vi "cross_talk).vi"(9 "Array":u8[](array[numeric]), 10 "Rising Index 2":i32[](array[numeric]), 11 "Rising Index":i32[](array[numeric])) -> (0 "data 2":cluster{"x":dbl, "y":dbl}[](array[cluster]) {"y" format="%.2f"; "x" format="%.2f"}, 1 "data":cluster{"x":dbl, "y":dbl}[](array[cluster]) {"y" format="%.2f"; "x" format="%.2f"}, 2 "x/y 2":dbl, 3 "x/y":dbl)   [LabVIEW 2012]
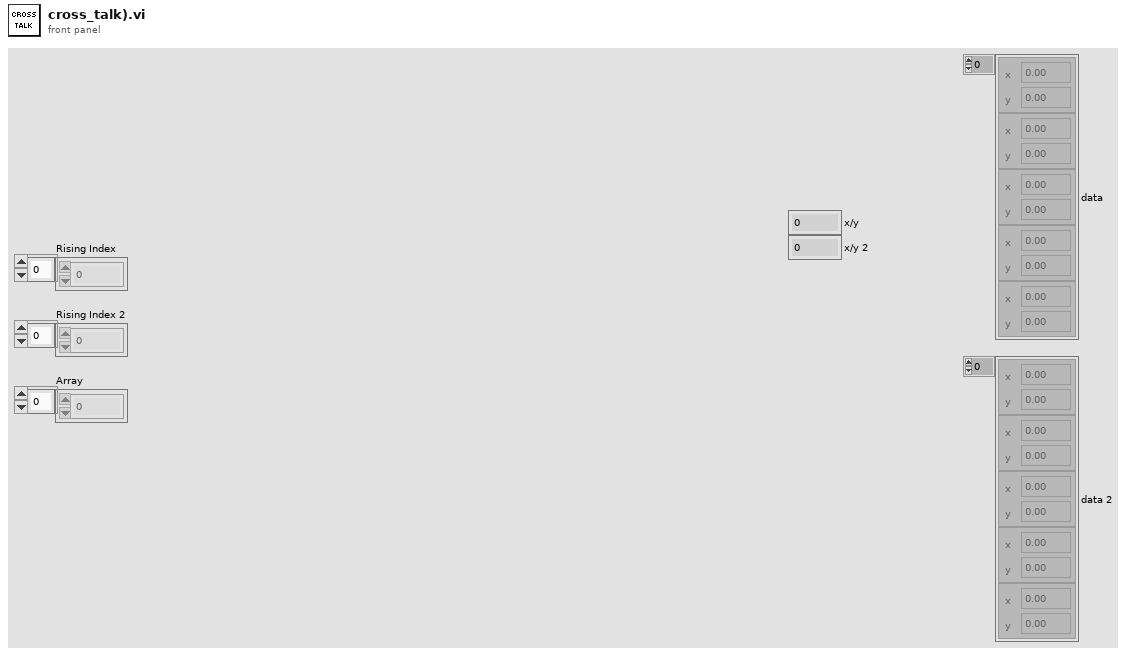
[diagram p1: front panel]
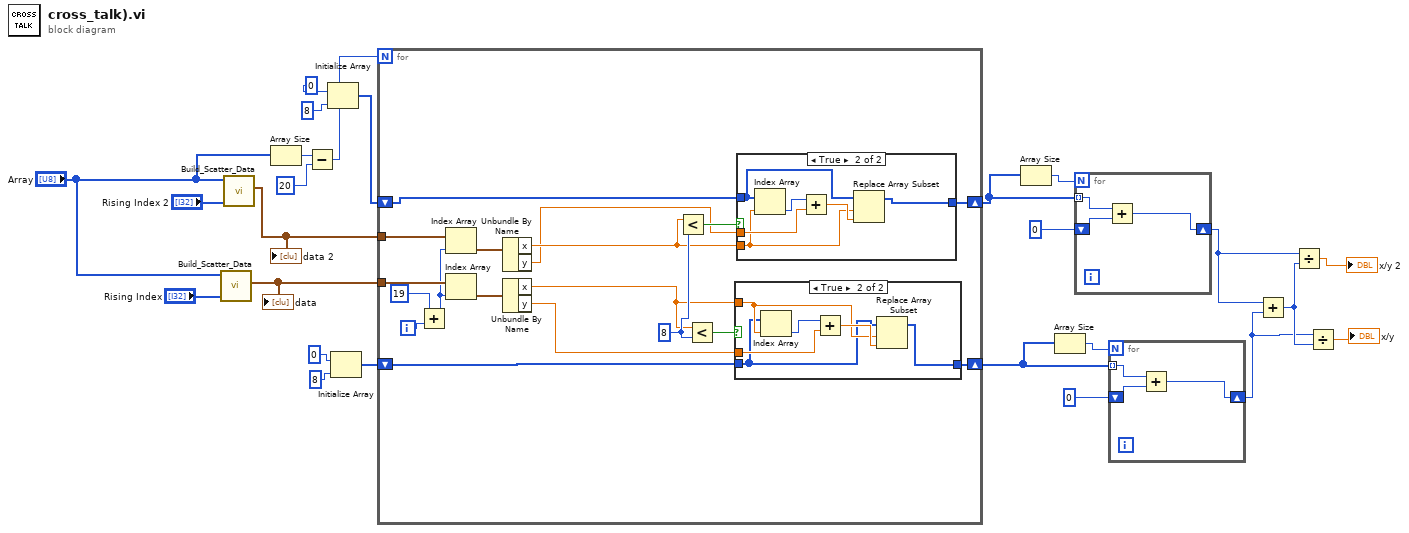
[diagram p0: block diagram]
diagram:
  n1 = call "Build_Scatter_Data.vi"("Rising Index"="Rising Index", "PMT (AI 0)"="Array") -> ("data"=w18:cluster{"x":dbl, "y":dbl}[])  [unwired: 9 in]
  "data" <- w18
  n2 = call "Build_Scatter_Data.vi"("Rising Index"="Rising Index 2", "PMT (AI 0)"="Array") -> ("data"=w19:cluster{"x":dbl, "y":dbl}[])  [unwired: 9 in]
  "data 2" <- w19
  n3 = Array Size(array="Array") -> (size(s)=w22:i32)
  n4 = Subtract(x=w22, y=20) -> (x-y=w21:i32)
  n5 = Initialize Array(0, 8) -> (w12:i32[])
  n6 = Initialize Array(0, 8) -> (w16:i32[])
  n7 = for {
    N: w21 -> [_]
    tunnel: w19 -> [w41]
    tunnel: w18 -> [w40]
    shift-right: [w31] -> w6
    shift-left: w16 -> [w33]
    shift-right: [w28] -> w10
    shift-left: w12 -> [w30]
    i -> [w43]
    w34 = 8
    n8 = Add(x=19, y=w43) -> (x+y=w39:i32)
    n9 = Index Array(array=w41, index=w39) -> (element=w38:cluster{"x":dbl, "y":dbl})
    n10 = Index Array(array=w40, index=w39) -> (element=w37:cluster{"x":dbl, "y":dbl})
    n11 = Unbundle By Name(w38) -> ("x"=w29:dbl, "y"=w27:dbl)
    n12 = Unbundle By Name(w37) -> ("x"=w32:dbl, "y"=w26:dbl)
    n13 = Less?(x=w29, y=w34) -> (x < y?=w36:bool)
    n14 = Less?(x=w32, y=w34) -> (x < y?=w35:bool)
    n15 = case shown="True" w35 {
      tunnel: w33 -> [w44 w46]
      tunnel: w32 -> [_ w48]
      tunnel: w26 -> [_ w50]
      tunnel: [w44 w45] -> w31
      frame False {
      }
      frame True {
        n16 = Index Array(array=w46, index=w48) -> (element=w47:i32)
        n17 = Add(x=w47, y=w50) -> (x+y=w49:dbl)
        n18 = Replace Array Subset(array=w46, new element=w49, index=w48) -> (w45:i32[])
      }
    }
    n19 = case shown="True" w36 {
      tunnel: w30 -> [w51 w57]
      tunnel: w27 -> [_ w56]
      tunnel: w29 -> [_ w53]
      tunnel: [w51 w52] -> w28
      frame False {
      }
      frame True {
        n20 = Index Array(array=w57, index=w53) -> (element=w55:i32)
        n21 = Add(x=w55, y=w56) -> (x+y=w54:dbl)
        n22 = Replace Array Subset(array=w57, new element=w54, index=w53) -> (w52:i32[])
      }
    }
  }
  n23 = Array Size(array=w10) -> (size(s)=w11:i32)
  n24 = Array Size(array=w6) -> (size(s)=w8:i32)
  n25 = for {
    N: w11 -> [_]
    tunnel: w10 -> [w60] mode=indexing
    shift-right: [w58] -> w4
    shift-left: 0 -> [w59]
    n26 = Add(x=w60, y=w59) -> (x+y=w58:i32)
  }
  n27 = for {
    N: w8 -> [_]
    tunnel: w6 -> [w63] mode=indexing
    shift-right: [w61] -> w3
    shift-left: 0 -> [w62]
    n28 = Add(x=w63, y=w62) -> (x+y=w61:i32)
  }
  n29 = Add(x=w4, y=w3) -> (x+y=w5:i32)
  n30 = Divide(x=w4, y=w5) -> (x/y=→"x/y 2":dbl)
  n31 = Divide(x=w3, y=w5) -> (x/y=→"x/y":dbl)
